vi "断电保存变量.vi"() -> ()   [LabVIEW 2016, in "斯坦道多参数.lvlib"]
panel:
  in  "滤波次数":u32=5
  in  "orp":bool
  in  "orp标液1":dbl
  in  "电导率标液2":dbl
  in  "电导率标液1":dbl
  in  "pH标液2":dbl
  in  "pH标液1":dbl
  in  "自动断线重连":bool=TRUE
  in  "藻密度":bool
  in  "连接方式":u16(ring) items=["Modbus RTU", "Modbus TCP"]
  in  "IP":string="localhost" caption="IP:"
  in  "Port":u16=502 caption="Port:"
  in  "定时控制输入":T1
  in  "探头选择":T2={"pH探头选择"=1, "DO探头选择"=0, "电导率探头选择"=1, "浊度探头选择"=0, "叶绿素a探头选择"=2, "蓝绿藻探头选择"=2, "orp探头选择"=1} {"orp探头选择" items=["禹山", "国弘", "纳清"]; "蓝绿藻探头选择" items=["禹山", "国弘", "纳清"]; "叶绿素a探头选择" items=["禹山", "国弘", "纳清"]; "浊度探头选择" items=["禹山", "国弘", "纳清"]; "电导率探头选择" items=["禹山", "国弘", "纳清"]; "DO探头选择" items=["禹山", "国弘", "纳清"]; "pH探头选择" items=["禹山", "国弘", "纳清"]}
  in  "蓝绿藻":bool
  in  "盐度自动获取":bool=TRUE
  out "大气压补偿":dbl=101.35
  out "盐度补偿":dbl
  in  "浊度标液2":dbl
  in  "浊度标液1":dbl
  in  "DO标液2":dbl=100.0
  in  "DO标液1":dbl
  in  "叶绿素a标液2":dbl
  in  "叶绿素a标液1":dbl
  in  "pH温度偏移补偿":dbl
  in  "Turb温度偏移补偿":dbl
  in  "Cond温度偏移补偿":dbl
  in  "DO温度偏移补偿":dbl
  in  "水样测定时间":dbl=5.0
  in  "叶绿素a启用":bool
  in  "标样核查配置":T3={"数据保存间隔"=1.0, "水温标样值"=0.0, "pH标样值"=0.0, "溶解氧标样值"=0.0, "电导率标样值"=0.0, "浊度标样值"=0.0}
  in  "Temp":bool
  in  "Cond":bool
  in  "Turb":bool
  in  "DO":bool
  in  "pH":bool
  in  "VISA资源名称":refnum<visa-resource-name>
  in  "水温通道":enum16{"pH", "Cond", "DO", "Turb"}(ring)
  # "请设置串口参数"
  # "请选择要启用的参数"
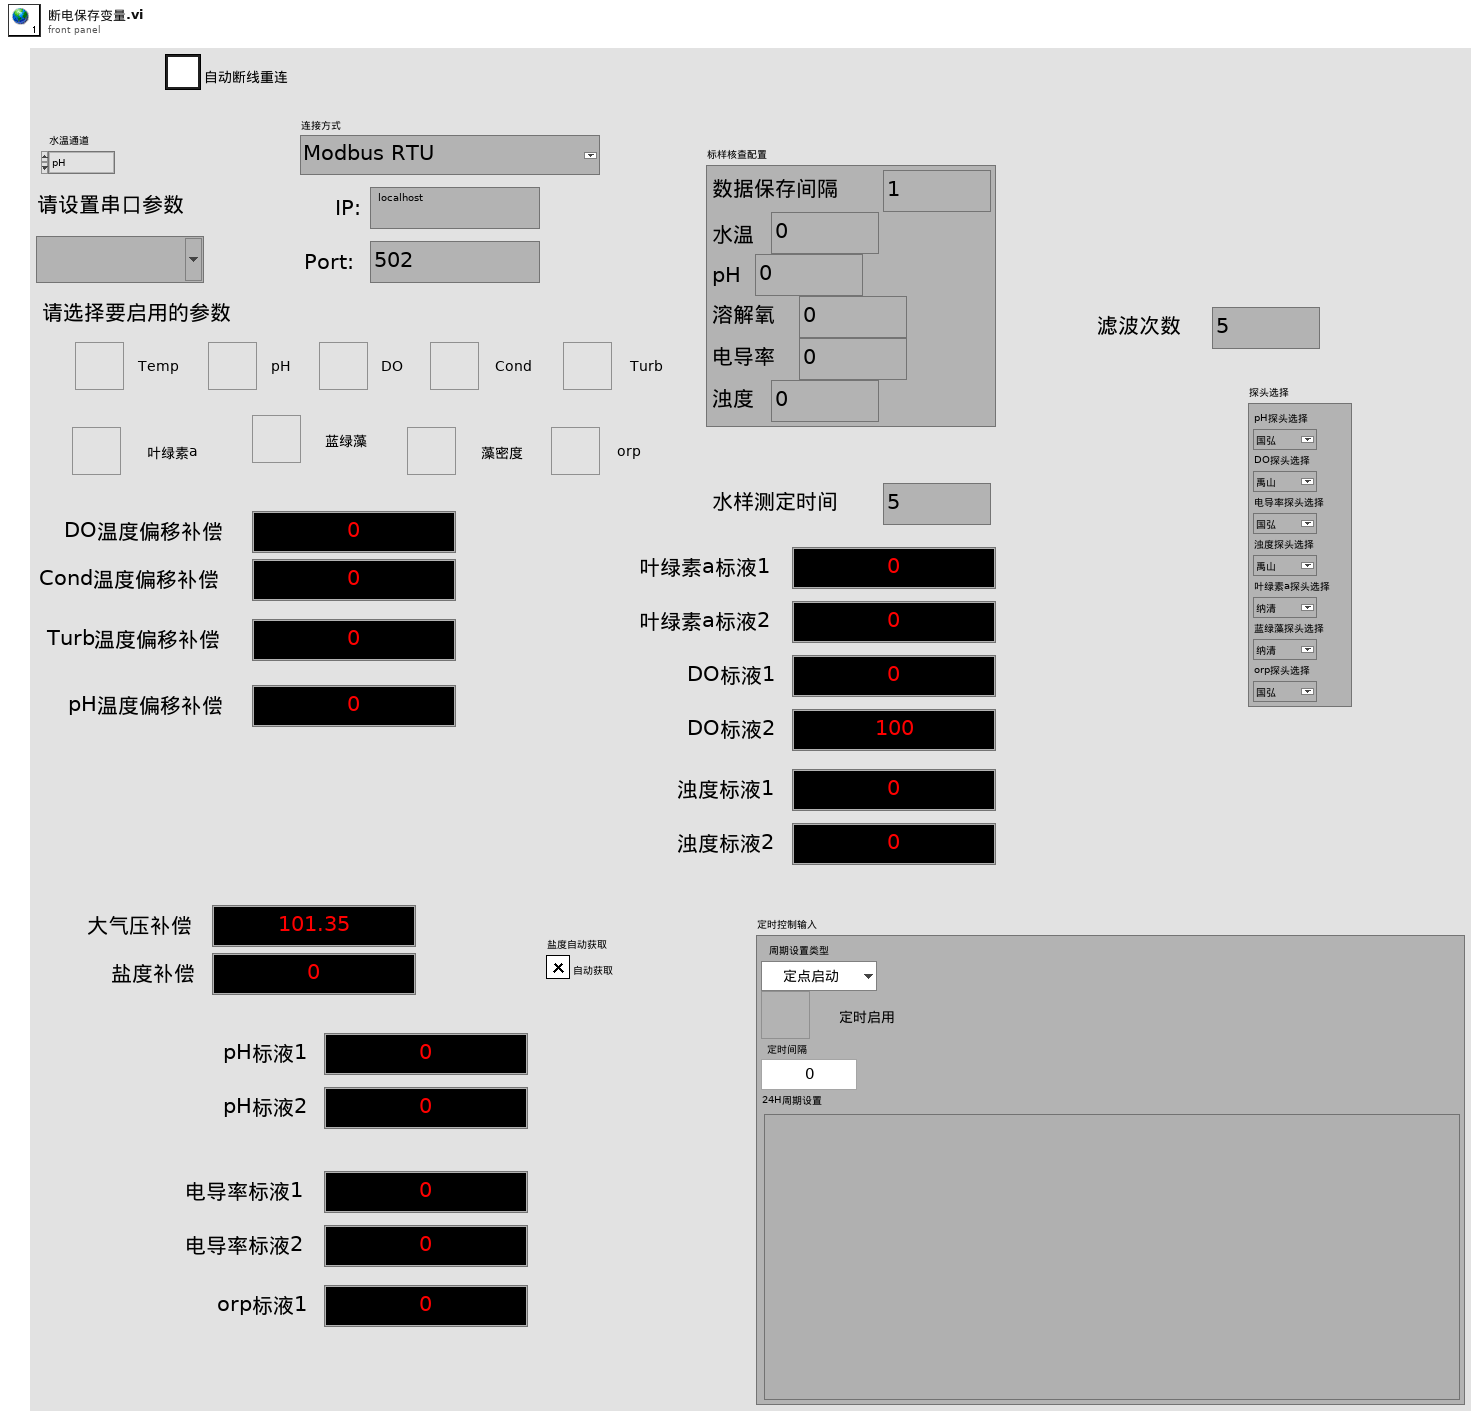
[diagram p1: front panel]
types:
  T1 = cluster{"周期设置类型":enum16{"定点启动", "间隔启动"}, "定时功能启用":bool, "定时间隔":u32, "24H周期设置":bool[]}
  T2 = cluster{"pH探头选择":u16, "DO探头选择":u16, "电导率探头选择":u16, "浊度探头选择":u16, "叶绿素a探头选择":u16, "蓝绿藻探头选择":u16, "orp探头选择":u16}
  T3 = cluster{"数据保存间隔":dbl, "水温标样值":dbl, "pH标样值":dbl, "溶解氧标样值":dbl, "电导率标样值":dbl, "浊度标样值":dbl}
diagram:
